vi "VITree.vi"   [LabVIEW 2014, in "Sixpack - Driver.lvlib"]
uses:
  Sixpack - Driver.lvlib
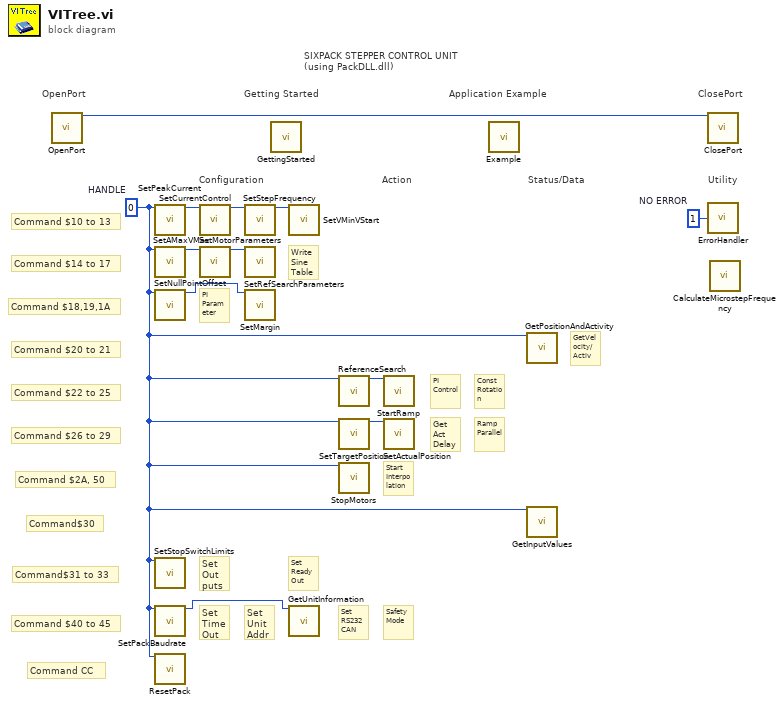
[diagram p0: block diagram]
diagram:
  w1 = i8 1  # NO ERROR
  w3 = 0  # HANDLE
  # "Command$31 to 33"
  # "ClosePort"
  # "OpenPort"
  # "Safety\nMode"
  # "Set\nRS232\nCAN"
  # "Command$30"
  # "Command $20 to 21"
  # "Application Example"
  # "Getting Started"
  # "SIXPACK STEPPER CONTROL UNIT\n(using PackDLL.dll)"
  # "Start\nInterpolation"
  # "Utility"
  # "Status/Data"
  # "Action"
  # "Set\nReady\nOut"
  # "Set\nUnit\nAddr"
  # "Set\nTime\nOut"
  # "Command CC"
  # "Command $40 to 45"
  # "Set\nOut\nputs"
  # "Command $2A, 50"
  # "Get\nAct\nDelay"
  # "Ramp\nParallel"
  # "Command $26 to 29"
  # "Const Rotation"
  # "PI\nControl"
  # "Command $22 to 25"
  # "GetVelocity/Activ"
  # "PI\nParameter"
  # "Command $18,19,1A"
  # "Write\nSine\nTable"
  # "Command $14 to 17"
  # "Configuration"
  # "Command $10 to 13"
  n1 = call "OpenPort.vi"() -> ("handle"=w12:i32)  [unwired: 18 in, 1 out]
  n2 = call "SetPeakCurrent.vi"("handle in"=w3) -> ("handle out"=w11:i32)  [unwired: 17 in, 1 out]
  n3 = call "SetAMaxVMax.vi"("handle in"=w3) -> ("handle out"=w8:i32)  [unwired: 17 in, 1 out]
  n4 = call "SetNullPointOffset.vi"("handle in"=w3) -> ("handle out"=w6:i32)  [unwired: 17 in, 1 out]
  n5 = call "SetStopSwitchLimits.vi"("handle in"=w3) -> ()  [unwired: 17 in, 2 out]
  n6 = call "SetPackBaudrate.vi"("handle in"=w3) -> ("handle out"=w2:i32)  [unwired: 17 in, 1 out]
  n7 = call "ResetPack.vi"("handle in"=w3) -> ()  [unwired: 17 in, 2 out]
  n8 = call "SetCurrentControl.vi"("handle in"=w11) -> ("handle out"=w10:i32)  [unwired: 17 in, 1 out]
  n9 = call "SetMotorParameters.vi"("handle in"=w8) -> ("handle out"=w7:i32)  [unwired: 17 in, 1 out]
  n10 = call "SetStepFrequency.vi"("handle in"=w10) -> ("handle out"=w9:i32)  [unwired: 17 in, 1 out]
  n11 = call "SetRefSearchParameters.vi"("handle in"=w7) -> ()  [unwired: 17 in, 2 out]
  n12 = call "SetMargin.vi"("handle in"=w6) -> ()  [unwired: 17 in, 2 out]
  n13 = call "GettingStarted.vi"() -> ()  [unwired: 1 in]
  n14 = call "SetVMinVStart.vi"("handle in"=w9) -> ()  [unwired: 17 in, 2 out]
  n15 = call "GetUnitInformation.vi"("handle in"=w2) -> ()  [unwired: 13 in, 6 out]
  n16 = call "ReferenceSearch.vi"("handle in"=w3) -> ("handle out"=w5:i32)  [unwired: 17 in, 1 out]
  n17 = call "SetTargetPosition.vi"("handle in"=w3) -> ("handle out"=w4:i32)  [unwired: 17 in, 1 out]
  n18 = call "StopMotors.vi"("handle in"=w3) -> ()  [unwired: 17 in, 2 out]
  n19 = call "StartRamp.vi"("handle in"=w5) -> ()  [unwired: 17 in, 2 out]
  n20 = call "SetActualPosition.vi"("handle in"=w4) -> ()  [unwired: 17 in, 2 out]
  n21 = call "Example.vi"() -> ()  [unwired: 1 in]
  n22 = call "GetPositionAndActivity.vi"("handle in"=w3) -> ()  [unwired: 14 in, 5 out]
  n23 = call "GetInputValues.vi"("handle in"=w3) -> ()  [unwired: 13 in, 6 out]
  n24 = call "ClosePort.vi"("handle"=w12) -> ()  [unwired: 19 in]
  n25 = call "ErrorHandler.vi"("BOOLEAN"=w1) -> ()  [unwired: 1 out]
  n26 = call "CalculateMicrostepFrequency.vi"() -> ()  [unwired: 3 in, 1 out]
